vi "ClientSerial.vi"() -> ()   [LabVIEW 2020]
uses:
  lib/SnapMB.lvlib
panel:
  out "Connection":i32
  in  "Format":enum32{"RTU", "ASCII"}(ring)
  in  "Flow":enum32{"NONE", "RTS/CTS"}(ring)
  in  "Stop Bits":i32(ring)=1 items=["1"=1, "2"=2]
  in  "Data Bits":i32(ring)=8 items=["7"=7, "8"=8]
  in  "Parity":string(combo)="E"
  in  "ComPort":string(combo)="COM3"
  in  "Baudrate":i32(ring)=19200 items=["4800"=4800, "9600"=9600, "19200"=19200, "38400"=38400, "57600"=57600, "115200"=115200]
  out "Write":string="No Error"
  in  "Write Start":u16=17
  out "Read":string="No Error"
  in  "Scan time (ms)":u32=500
  out "JobTime (ms)":i32
  out "Connected":bool
  out "error out":errorcluster
  out "Run":bool
  in  "?":bool
  in  "Amount":u16=16
  in  "Read Start":u16=1
  out "RD Data":u16[](array[numeric]) format="%x"
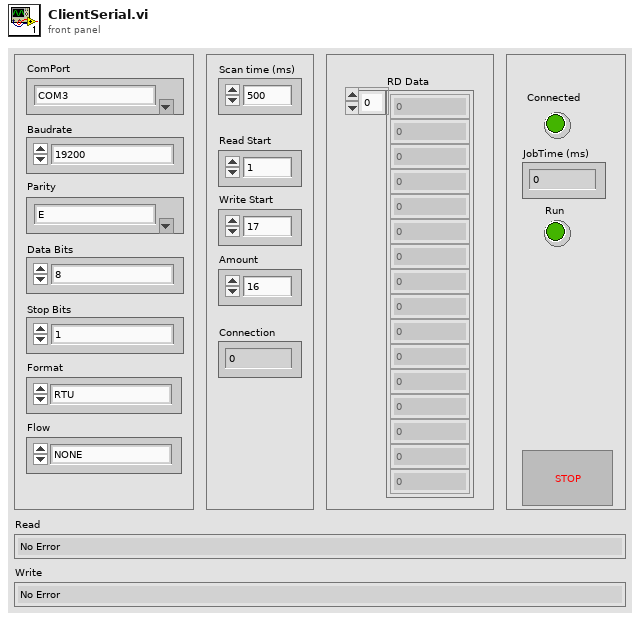
[diagram p1: front panel]
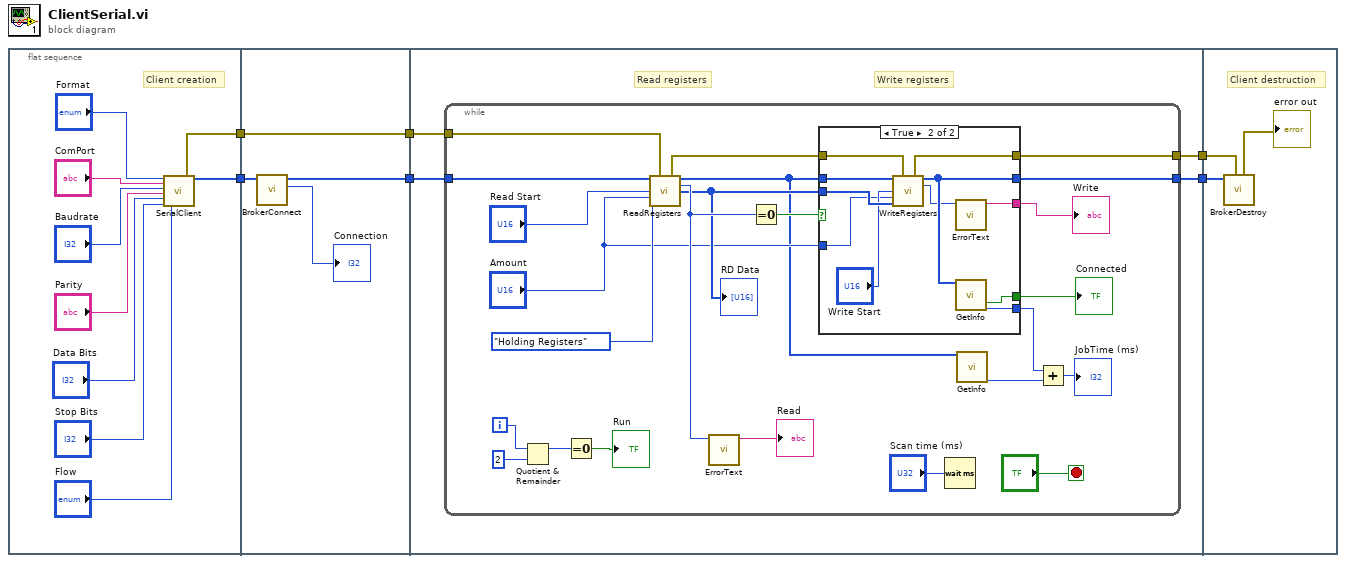
[diagram p0: block diagram]
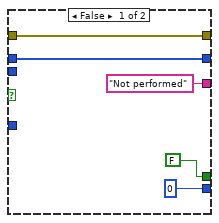
[diagram p2: hidden frame]
diagram:
  n1 = flat-sequence {
    tunnel: [w14] -> w4
    tunnel: [w15] -> w3
    tunnel: w4 -> [w17]
    tunnel: w3 -> [w19]
    tunnel: [w19] -> w2
    tunnel: [w18] -> w1
    tunnel: w2 -> [w22]
    tunnel: [w21] -> w6
    tunnel: [w20] -> w5
    tunnel: w1 -> [w23]
    tunnel: w6 -> [w65]
    tunnel: w5 -> [w64]
    frame #0 {
      # "Client creation"
      n2 = call "SerialClient.vi"("Format"="Format", "Port"="ComPort", "Baudrate"="Baudrate", "Parity"="Parity", "Data Bits"="Data Bits", "Stop Bits"="Stop Bits", "Flow"="Flow") -> ("error out"=w15:errorcluster, "Handle Out"=w14:u64[])  [unwired: 11 in]
    }
    frame #1 {
      n3 = call "BrokerConnect.vi"("Handle In"=w17) -> ("Result"=→"Connection":i32, "Handle Out"=w18:u64[])  [unwired: 8 in, 1 out]
    }
    frame #2 {
      # "Write registers"
      # "Read registers"
      n4 = while {
        tunnel: w23 -> [w42]
        tunnel: w22 -> [w41]
        tunnel: [w31] -> w21
        tunnel: [w29] -> w20
        i -> [w47]
        stop <- "?" stop-if-true
        n5 = Quotient & Remainder(x=w47, y=2) -> (x-y*floor(x/y)=w45:i32)  [unwired: 1 out]
        n6 = Equal To 0?(x=w45) -> (x = 0?=→"Run":bool)
        n7 = call "ReadRegisters.vi"("Handle In"=w42, "error in (no error)"=w41, "Read Start"="Read Start", "Read Amount"="Amount", "Area"=enum16{"Holding Registers", "Input Registers"}."Holding Registers") -> ("error out"=w30:errorcluster, "Handle Out"=w32:u64[], "Result"=w35:i32, "RD Data"=w34:u16[])  [unwired: 7 in]
        "RD Data" <- w34
        n8 = call "ErrorText.vi"("ErrNo"=w35) -> ("ErrMessage"=→"Read":string)  [unwired: 9 in, 1 out]
        n9 = Equal To 0?(x=w35) -> (x = 0?=w36:bool)
        n10 = case shown="True" w36 {
          tunnel: w32 -> [w51 w63]
          tunnel: w34 -> [_ w62]
          tunnel: "Amount" -> [_ w60]
          tunnel: [w51 w57] -> w31
          tunnel: w30 -> [w52 w59]
          tunnel: [w52 w58] -> w29
          tunnel: [0 ("JobTime") w56] -> w27
          tunnel: [FALSE ("Connected") w55] -> w25
          tunnel: ["Not performed" ("ErrMessage") w54] -> w24
          frame False {
          }
          frame True {
            n11 = call "WriteRegisters.vi"("Handle In"=w63, "error in (no error)"=w59, "Write Start"="Write Start", "Write Amount"=w60, "WR Data"=w62) -> ("error out"=w58:errorcluster, "Handle Out"=w57:u64[], "Result"=w53:i32)  [unwired: 7 in, 1 out]
            n12 = call "ErrorText.vi"("ErrNo"=w53) -> ("ErrMessage"=w54:string)  [unwired: 9 in, 1 out]
            n13 = call "GetInfo.vi"("Broker In"=w57) -> ("Connected"=w55:bool, "JobTime"=w56:i32)  [unwired: 12 in, 5 out]
          }
        }
        "Connected" <- w25
        "Write" <- w24
        n14 = Wait (ms)(milliseconds to wait="Scan time (ms)") -> ()  [unwired: 1 out]
        n15 = call "GetInfo.vi"("Broker In"=w32) -> ("JobTime"=w26:i32)  [unwired: 12 in, 6 out]
        n16 = Add(x=w27, y=w26) -> (x+y=→"JobTime (ms)":i32)
      }
    }
    frame #3 {
      # "Client destruction"
      n17 = call "BrokerDestroy.vi"("error in (no error)"=w64, "Handle In"=w65) -> ("error out"=→"error out":errorcluster)  [unwired: 9 in]
    }
  }
